vi "Car Wash.vi"() -> ()   [LabVIEW 2024]
uses:
  Controls/Car Wash Indicators.ctl
  Controls/Wash Options.ctl
  Controls/DataCluster.ctl
  <vilib>/Utility/error.llb/Error Cluster From Error Code.vi
  <vilib>/ErrorRing/Error Ring.xnode
panel:
  out "Error Out":errorcluster
  in  "Error In":errorcluster
  in  "Start":bool
  out "Elapsed Time":dbl format="%0.2f"
  in  "stop":bool
  out "Wash Entry":bool
  in  "Wash Options":T1
  in  "Car Position Slider":u8(slide) max=3 scale=0.0..4.0
  out "Car Wash Indicators":T2
  # "Entry Console"
  # "Car Wash Display"
  # "Car Position Simulation"
  # "Pre-Soak\nH-P Wash\nL-P Wax\nSpot Free Rinse"
  # "Underbody Wash\nBug Remover"
  # "Tire Shine\nAir Dry"
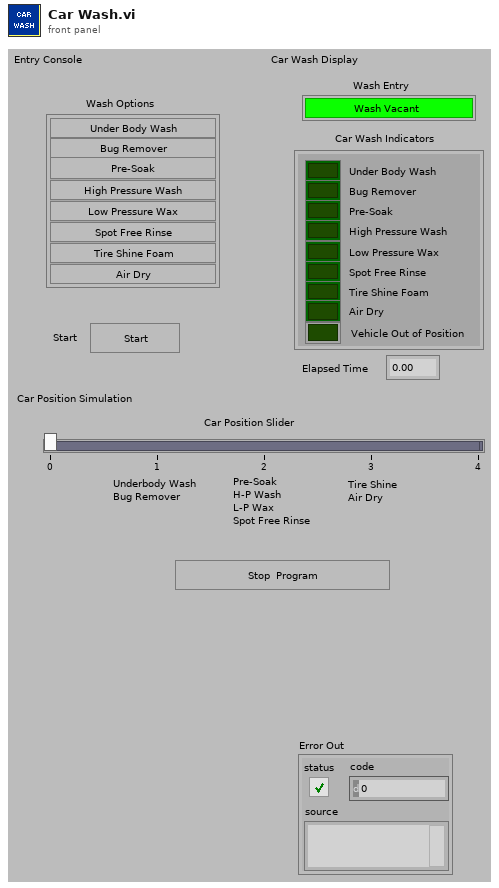
[diagram p1: front panel]
types:
  T1 = typedef "Wash Options.ctl" = cluster{"Underbody Wash":bool, "Bug Remover":bool, "Pre-Soak":bool, "High Pressure Wash":bool, "Low Pressure Wax":bool, "Spot Free Rinse":bool, "Tire Shine Foam":bool, "Air Dry":bool}
  T2 = typedef "Car Wash Indicators.ctl" = cluster{"Under Body Wash":bool, "Bug Remover":bool, "Pre-Soak":bool, "High Pressure Wash":bool, "Low Pressure Wax":bool, "Spot Free Rinse":bool, "Tire Shine Foam":bool, "Air Dry":bool, "Vehicle Out of Position":bool}
  T3 = enum16{"Create", "Enqueue", "Dequeue", "Enstack", "Flush", "Clear"}
  T4 = enum8{"Enabled", "Disabled", "Disabled and Grayed Out"}
  T5 = typedef "DataCluster.ctl" = cluster{"Wash Options":T1, "Elapsed Time (s)":dbl, "Car Wash Indicators":T2, "Wash Entry":bool, "Wash Running":bool, "Sorted Wash ":enum16{"Under Body Wash", "Bug Remover", "Pre-Soak", "High Pressure Wash", "Low Pressure Wax", "Spot Free Rinse", "Tire Shine Foam", "Air Dry", "Skip"}[], "Timer Elapsed?":bool, "Time Target (s)":dbl}
  T6 = enum16{"Under Body Wash", "Bug Remover", "Pre-Soak", "High Pressure Wash", "Low Pressure Wax", "Spot Free Rinse", "Tire Shine Foam", "Air Dry", "Skip"}[]
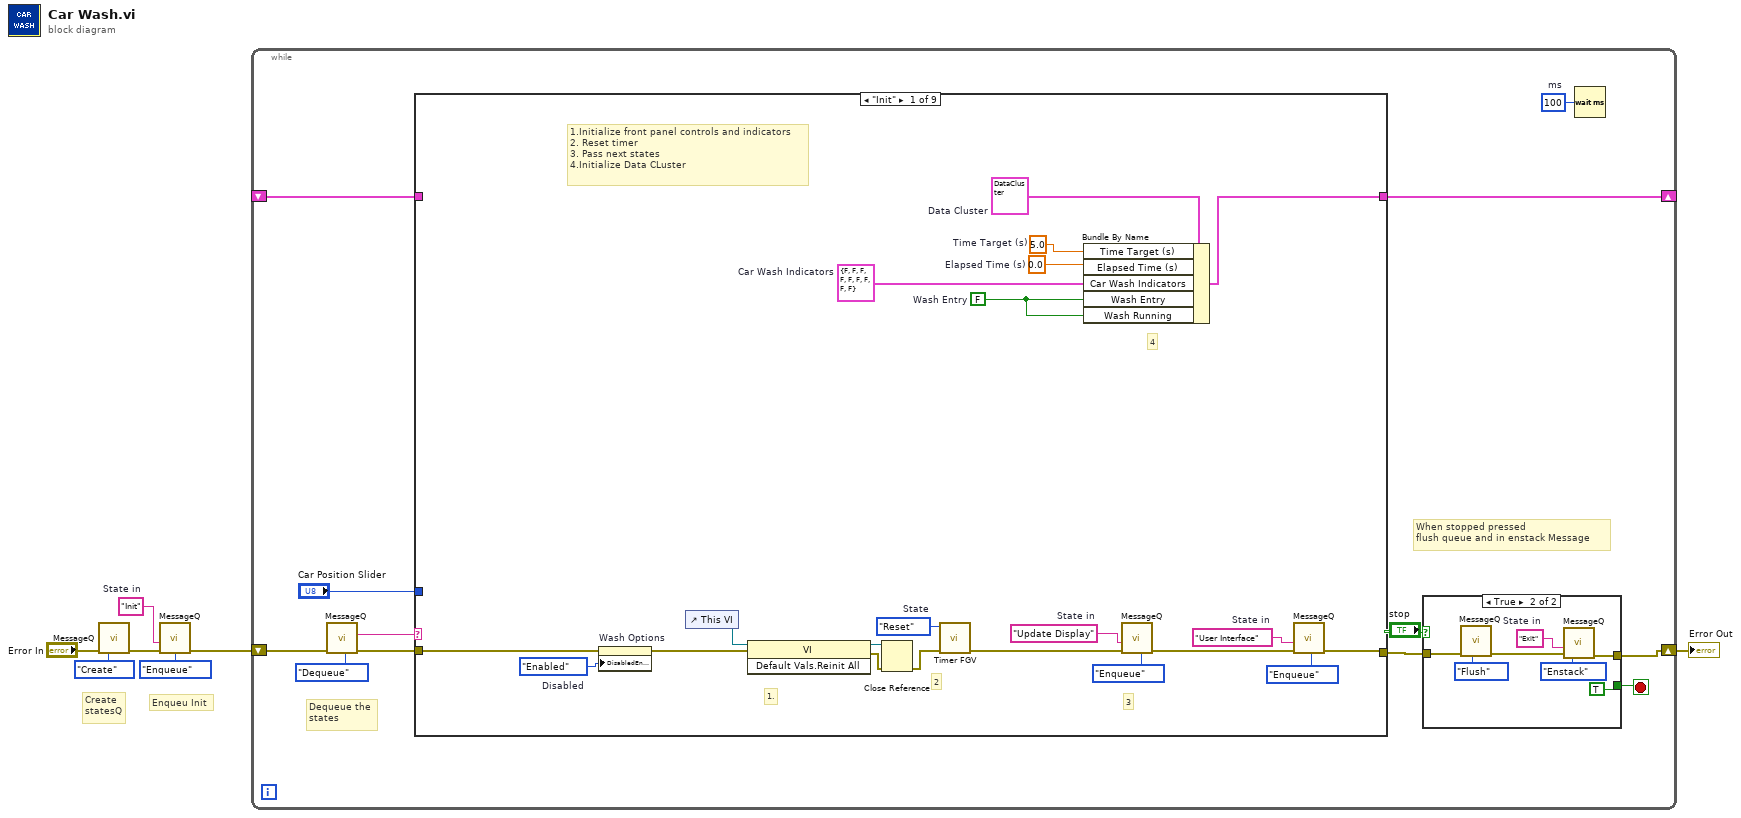
[diagram p0: block diagram]
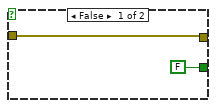
[diagram p2: hidden frame]
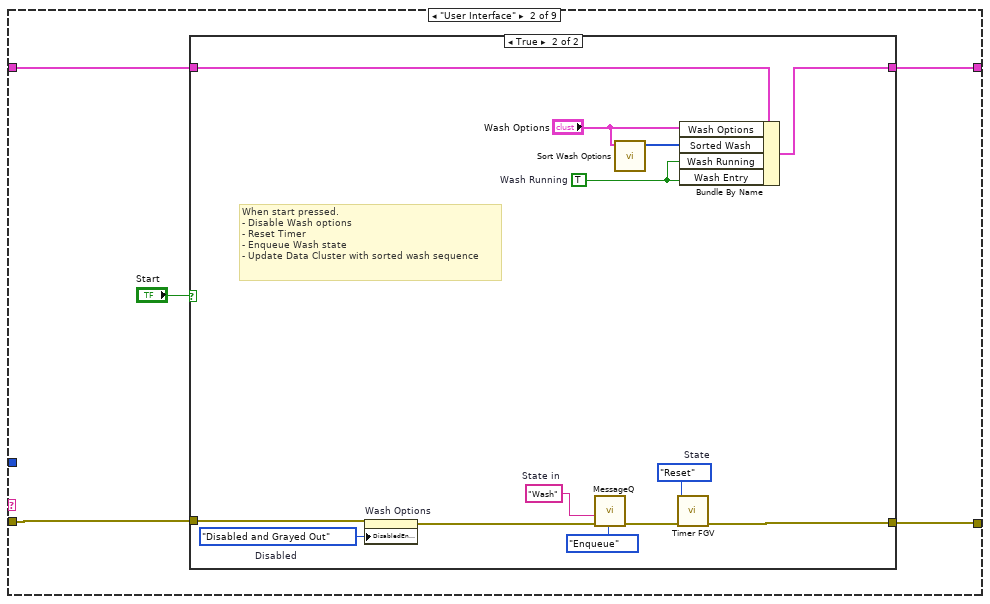
[diagram p3: hidden frame]
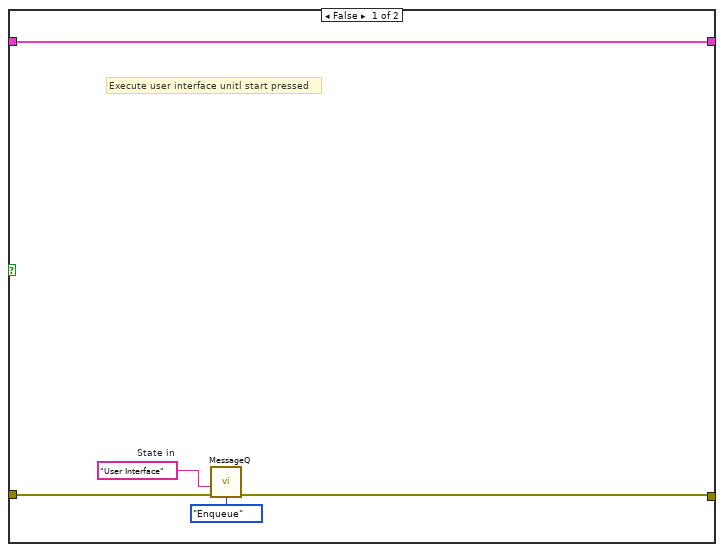
[diagram p4: hidden frame]
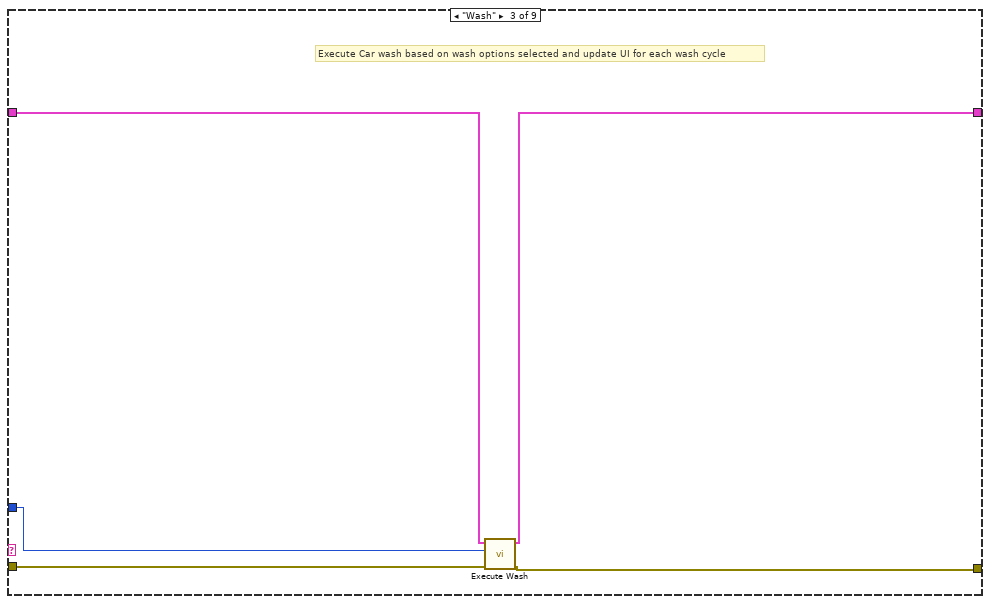
[diagram p5: hidden frame]
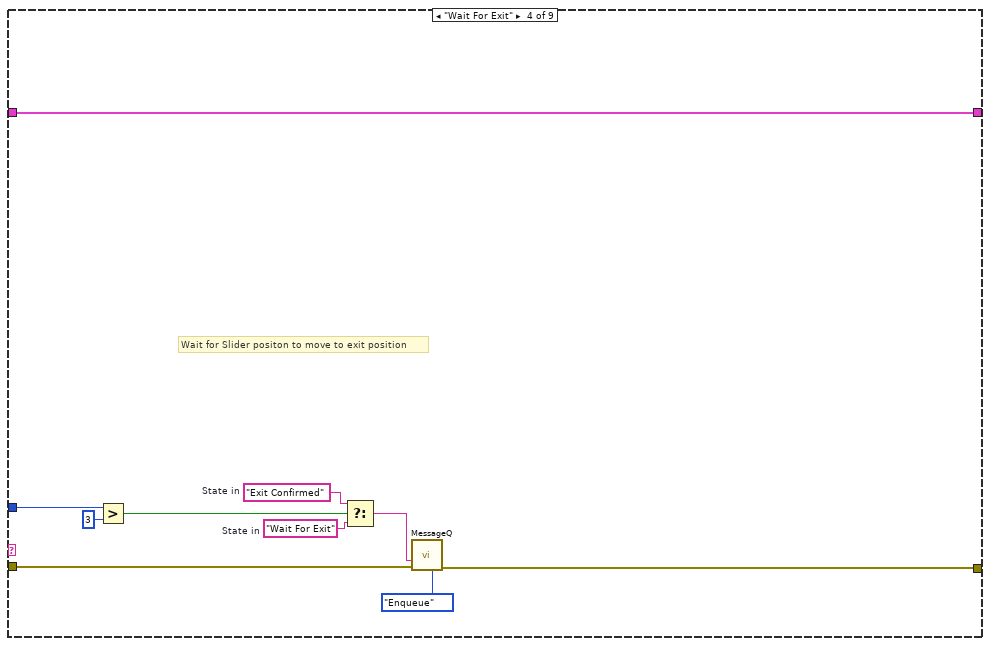
[diagram p6: hidden frame]
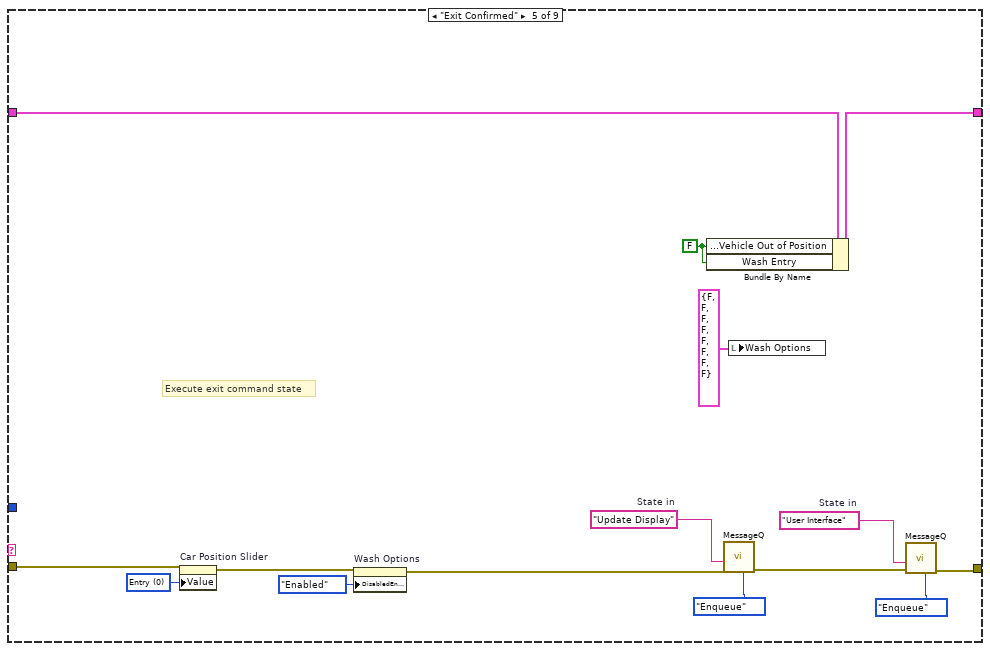
[diagram p7: hidden frame]
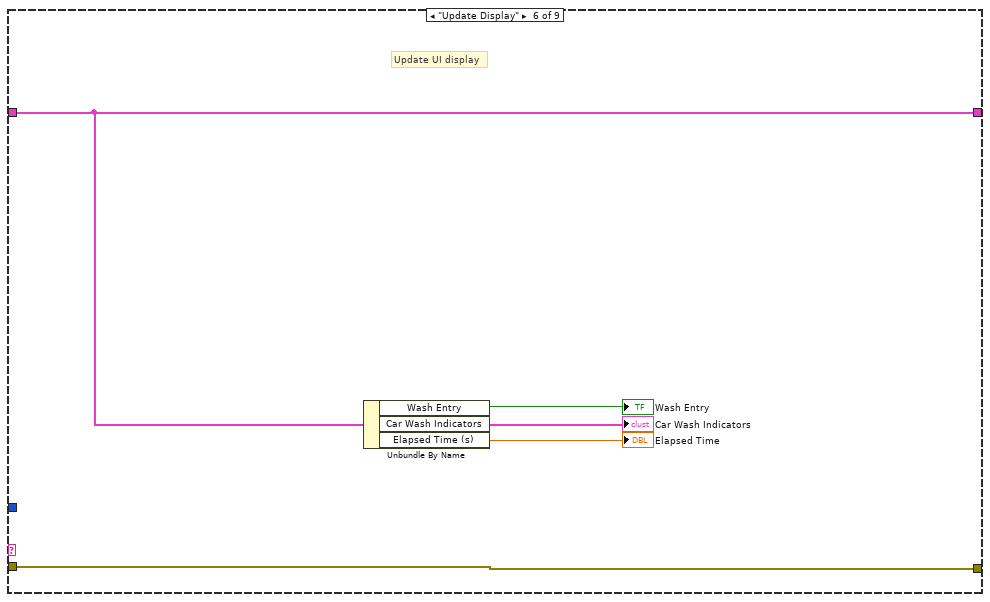
[diagram p8: hidden frame]
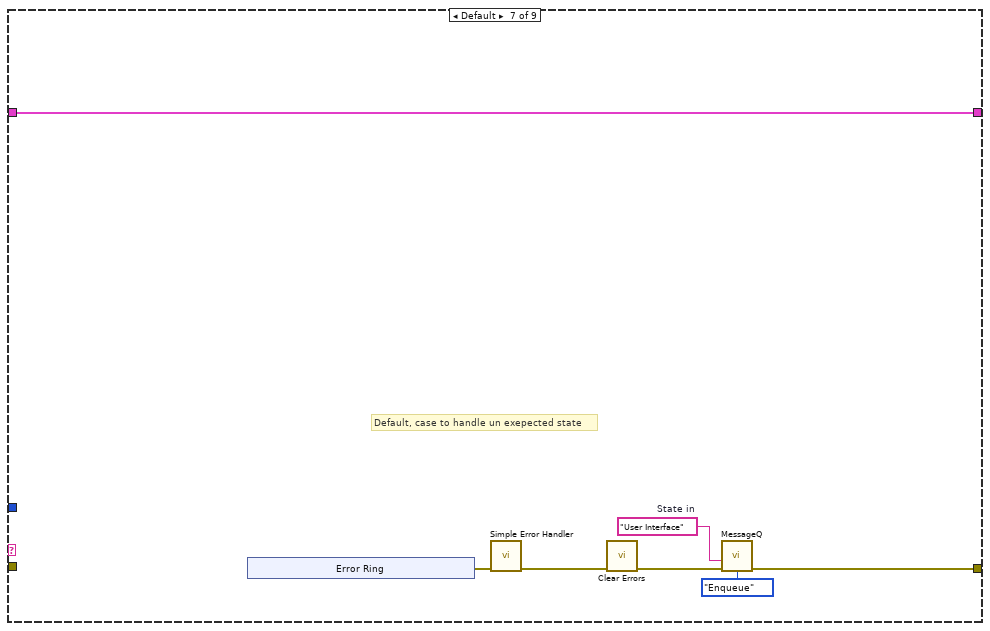
[diagram p9: hidden frame]
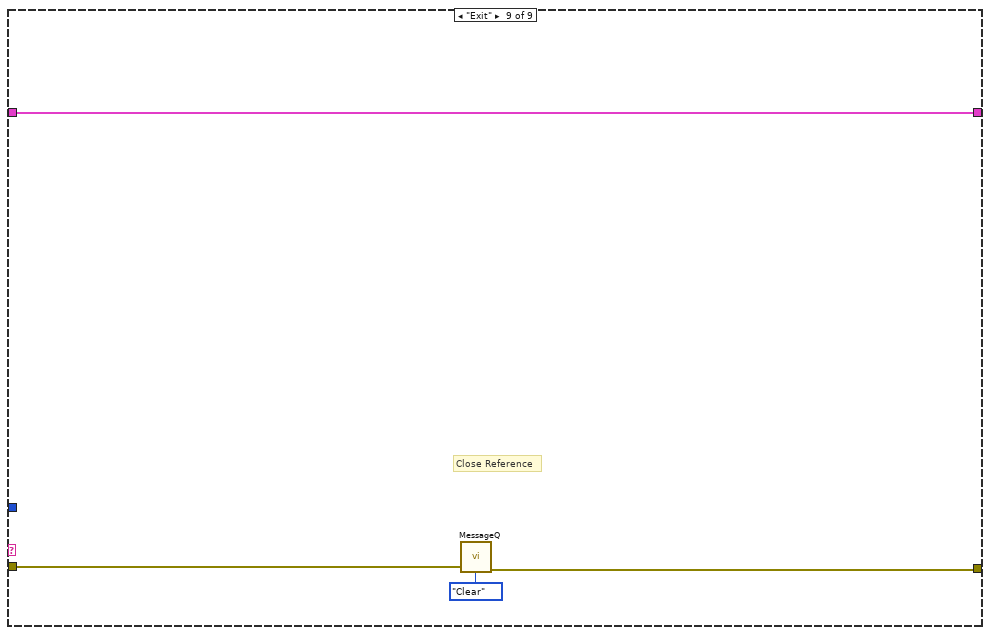
[diagram p11: hidden frame]
diagram:
  w3 = "Init"  # State in
  # "Enqueu Init"
  # "Create\nstatesQ"
  n1 = call "MessageQ.vi"("Error In"="Error In", "QState"=T3."Create") -> ("Error Out"=w4:errorcluster)  [unwired: 8 in, 1 out]
  n2 = call "MessageQ.vi"("Error In"=w4, "State in"=w3, "QState"=T3."Enqueue") -> ("Error Out"=w2:errorcluster)  [unwired: 7 in, 1 out]
  n3 = while {
    shift-right: [w10] -> w1
    shift-left: w2 -> [w19]
    shift-right: [w16] -> _
    shift-left: _ -> [w15]
    stop <- w9 stop-if-true
    w8 = u32 100  # ms
    # "When stopped pressed\nflush queue and in enstack Message"
    # "Dequeue the\nstates"
    n4 = call "MessageQ.vi"("Error In"=w19, "QState"=T3."Dequeue") -> ("Error Out"=w17:errorcluster, "State Out"=w18:string)  [unwired: 8 in]
    n5 = case shown="\"Init\"" w18 {
      tunnel: w17 -> [w44 w52 w74 w86 w98 w107 _ w120 w123]
      tunnel: [w46 w53 w76 w85 w90 w106 w114 w121 w125] -> w16
      tunnel: w15 -> [_ w54 w77 w85 w94 w106 w114 w121 w125]
      tunnel: [w40 w51 w73 w87 w102 w107 w109 w120 w122] -> w11
      tunnel: "Car Position Slider" -> [_ _ w75 w84 _ _ _ _ _]
      frame "Init" {
        w29 = 5.0  # Time Target (s)
        w36 = "User Interface"  # State in
        w37 = "Update Display"  # State in
        w43 = enum16{"Reset", "Read", "Pause"}."Reset"  # State
        w45 = T4."Enabled"  # Disabled
        w47 = 0.0  # Elapsed Time (s)
        w48 = T2 {"Under Body Wash"=FALSE, "Bug Remover"=FALSE, "Pre-Soak"=FALSE, "High Pressure Wash"=FALSE, "Low Pressure Wax"=FALSE, "Spot Free Rinse"=FALSE, "Tire Shine Foam"=FALSE, "Air Dry"=FALSE, "Vehicle Out of Position"=FALSE}  # Car Wash Indicators
        w35 = FALSE  # Wash Entry
        w49 = T5 {"Wash Options"={"Underbody Wash"=FALSE, "Bug Remover"=FALSE, "Pre-Soak"=FALSE, "High Pressure Wash"=FALSE, "Low Pressure Wax"=FALSE, "Spot Free Rinse"=FALSE, "Tire Shine Foam"=FALSE, "Air Dry"=FALSE}, "Elapsed Time (s)"=0.0, "Car Wash Indicators"={"Under Body Wash"=FALSE, "Bug Remover"=FALSE, "Pre-Soak"=FALSE, "High Pressure Wash"=FALSE, "Low Pressure Wax"=FALSE, "Spot Free Rinse"=FALSE, "Tire Shine Foam"=FALSE, "Air Dry"=FALSE, "Vehicle Out of Position"=FALSE}, "Wash Entry"=FALSE, "Wash Running"=FALSE, "Sorted Wash "=[], "Timer Elapsed?"=FALSE, "Time Target (s)"=0.0}  # Data Cluster
        # "4"
        # "3"
        # "2"
        # "1."
        # "1.Initialize front panel controls and indicators\n2. Reset timer\n3. Pass next states\n4.Initialize Data CLuster"
        n6 = property on="Wash Options" class="Clust (strict)"(error in=w44, "DisabledEnum"=w45) -> (error out=w32:errorcluster)  [unwired: 1 in, 1 out]
        n7 = control-ref of="This VI"() -> (w34:refnum<vi>)
        n8 = invoke class="VI" method="Default Vals.Reinit All"(reference=w34, error in=w32) -> (reference out=w33:refnum<vi>, error out=w31:errorcluster)  [unwired: 1 in, 1 out]
        n9 = Close Reference(reference=w33, error in (no error)=w31) -> (error out=w30:errorcluster)
        n10 = call "Timer FGV.vi"("Error In"=w30, "State"=w43) -> ("Error Out"=w42:errorcluster)  [unwired: 7 in, 2 out]
        n11 = Bundle By Name(cluster=w49, "Time Target (s)"=w29, "Elapsed Time (s)"=w47, "Car Wash Indicators"=w48, "Wash Entry"=w35, "Wash Running"=w35) -> (w46:T5)
        n12 = call "MessageQ.vi"("Error In"=w42, "State in"=w37, "QState"=T3."Enqueue") -> ("Error Out"=w41:errorcluster)  [unwired: 7 in, 1 out]
        n13 = call "MessageQ.vi"("Error In"=w41, "State in"=w36, "QState"=T3."Enqueue") -> ("Error Out"=w40:errorcluster)  [unwired: 7 in, 1 out]
      }
      frame "User Interface" {
        n14 = case shown="True" "Start" {
          tunnel: w54 -> [w59 w72]
          tunnel: [w59 w71] -> w53
          tunnel: w52 -> [w58 w70]
          tunnel: [w57 w69] -> w51
          frame False {
            w55 = "User Interface"  # State in
            # "Execute user interface unitl start pressed"
            n15 = call "MessageQ.vi"("Error In"=w58, "State in"=w55, "QState"=T3."Enqueue") -> ("Error Out"=w57:errorcluster)  [unwired: 7 in, 1 out]
          }
          frame True {
            w62 = enum16{"Reset", "Read", "Pause"}."Reset"  # State
            w63 = "Wash"  # State in
            w61 = TRUE  # Wash Running
            w68 = T4."Disabled and Grayed Out"  # Disabled
            # "When start pressed.\n- Disable Wash options\n- Reset Timer\n- Enqueue Wash state\n- Update Data Cluster with sorted wash sequence"
            n16 = property on="Wash Options" class="Clust (strict)"(error in=w70, "DisabledEnum"=w68) -> (error out=w66:errorcluster)  [unwired: 1 in, 1 out]
            n17 = call "MessageQ.vi"("Error In"=w66, "State in"=w63, "QState"=T3."Enqueue") -> ("Error Out"=w65:errorcluster)  [unwired: 7 in, 1 out]
            n18 = call "Sort Wash Options.vi"("Wash Options"="Wash Options") -> ("Sorted Wash"=w67:T6)  [unwired: 10 in]
            n19 = call "Timer FGV.vi"("Error In"=w65, "State"=w62) -> ("Error Out"=w69:errorcluster)  [unwired: 7 in, 2 out]
            n20 = Bundle By Name(cluster=w72, "Wash Options"="Wash Options", "Sorted Wash"=w67, "Wash Running"=w61, "Wash Entry"=w61) -> (w71:T5)
          }
        }
      }
      frame "Wash" {
        # "Execute Car wash based on wash options selected and update UI for each wash cycle"
        n21 = call "Execute Wash.vi"("Error In"=w74, "Car Position Slider"=w75, "Data Cluster"=w77) -> ("Error Out"=w73:errorcluster, "Data Cluster Out"=w76:T5)  [unwired: 7 in]
      }
      frame "Wait For Exit" {
        w80 = "Wait For Exit"  # State in
        w82 = "Exit Confirmed"  # State in
        # "Wait for Slider positon to move to exit position"
        n22 = Greater?(x=w84, y=u8 3) -> (0:w81:bool)
        n23 = Select(t=w82, s=w81, f=w80) -> (s? t:f=w78:string)
        n24 = call "MessageQ.vi"("Error In"=w86, "State in"=w78, "QState"=T3."Enqueue") -> ("Error Out"=w87:errorcluster)  [unwired: 7 in, 1 out]
      }
      frame "Exit Confirmed" {
        w93 = "Update Display"  # State in
        w89 = FALSE ("Car Wash Indicators.Vehicle Out of Position")
        w99 = u8 0 items=["Entry", "Station 1", "Station 2", "Station 3", "Exit"] ("Car Position Slider")
        w100 = "User Interface"  # State in
        # "Execute exit command state"
        n25 = property on="Car Position Slider" class="Slide (strict)"(error in=w98, "Value"=w99) -> (error out=w97:errorcluster)  [unwired: 1 in, 1 out]
        n26 = property on="Wash Options" class="Clust (strict)"(error in=w97, "DisabledEnum"=T4."Enabled" ("Disabled")) -> (error out=w95:errorcluster)  [unwired: 1 in, 1 out]
        n27 = Bundle By Name(cluster=w94, "Car Wash Indicators.Vehicle Out of Position"=w89, "Wash Entry"=w89) -> (w90:T5)
        n28 = call "MessageQ.vi"("Error In"=w95, "State in"=w93, "QState"=T3."Enqueue") -> ("Error Out"=w91:errorcluster)  [unwired: 7 in, 1 out]
        n29 = local write "Wash Options"(T1 {"Underbody Wash"=FALSE, "Bug Remover"=FALSE, "Pre-Soak"=FALSE, "High Pressure Wash"=FALSE, "Low Pressure Wax"=FALSE, "Spot Free Rinse"=FALSE, "Tire Shine Foam"=FALSE, "Air Dry"=FALSE} ("Wash Options")) -> ()
        n30 = call "MessageQ.vi"("Error In"=w91, "State in"=w100, "QState"=T3."Enqueue") -> ("Error Out"=w102:errorcluster)  [unwired: 7 in, 1 out]
      }
      frame "Update Display" {
        # "Update UI display"
        n31 = Unbundle By Name(w106) -> ("Wash Entry"=→"Wash Entry":bool, "Car Wash Indicators"=→"Car Wash Indicators":T2, "Elapsed Time (s)"=→"Elapsed Time":dbl)
      }
      frame Default {
        w108 = "User Interface"  # State in
        # "Default, case to handle un exepected state"
        n32 = xnode "Error Ring"() -> ("error out"=w113:errorcluster)
        n33 = call <vilib>:"Simple Error Handler.vi"("error in (no error)"=w113) -> ("error out"=w112:errorcluster)  [unwired: 4 in, 4 out]
        n34 = call <vilib>:"Clear Errors.vi"("error in (no error)"=w112) -> ("error out"=w110:errorcluster)  [unwired: 5 in, 1 out]
        n35 = call "MessageQ.vi"("Error In"=w110, "State in"=w108, "QState"=T3."Enqueue") -> ("Error Out"=w109:errorcluster)  [unwired: 7 in, 1 out]
      }
      frame "Error" {
        # "Handle the errors"
      }
      frame "Exit" {
        # "Close Reference"
        n36 = call "MessageQ.vi"("Error In"=w123, "QState"=T3."Clear") -> ("Error Out"=w122:errorcluster)  [unwired: 8 in, 1 out]
      }
    }
    n37 = case shown="True" "stop" {
      tunnel: w11 -> [w21 w24]
      tunnel: [w21 w23] -> w10
      tunnel: [FALSE TRUE] -> w9
      frame False {
      }
      frame True {
        w26 = "Exit"  # State in
        n38 = call "MessageQ.vi"("Error In"=w24, "QState"=T3."Flush") -> ("Error Out"=w25:errorcluster)  [unwired: 8 in, 1 out]
        n39 = call "MessageQ.vi"("Error In"=w25, "State in"=w26, "QState"=T3."Enstack") -> ("Error Out"=w23:errorcluster)  [unwired: 7 in, 1 out]
      }
    }
    n40 = Wait (ms)(milliseconds to wait=w8) -> ()  [unwired: 1 out]
  }
  "Error Out" <- w1
